vi "ErrorLogVI.vi"(8 "Error In":errorcluster, 11 "Station":string) -> ()   [LabVIEW 2017]
doc: "This VI log's Error to ErrLog.txt File.\nPath:- C:/.../Documents/VisionInsp folder in PC.\nChange Folder name If you want to save Error Log into Another Folder."
uses:
  <vilib>/Utility/sysdir.llb/System Directory Type.ctl
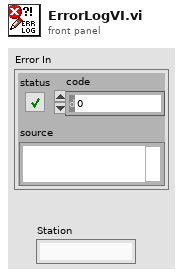
[diagram p1: front panel]
types:
  T1 = enum16{"open", "replace", "create", "open or create", "replace or create", "replace or create with confirmation"}
  T2 = typedef "System Directory Type.ctl" = i32
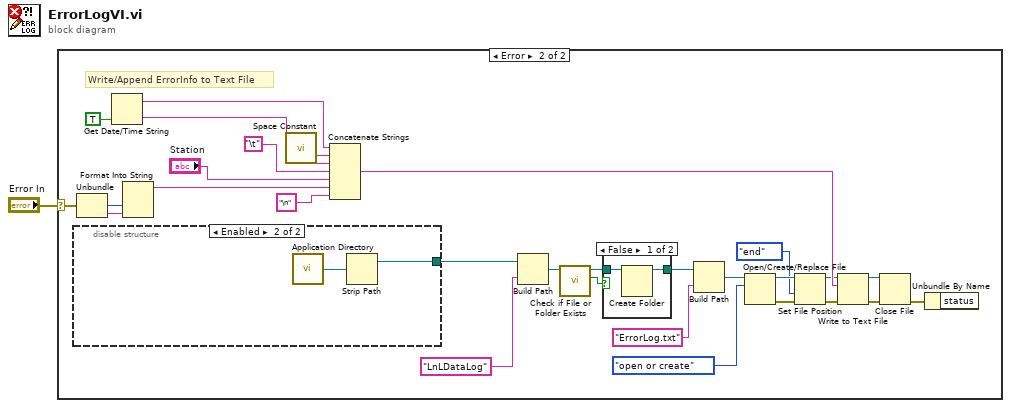
[diagram p0: block diagram]
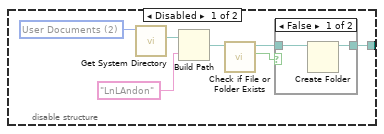
[diagram p3: hidden frame]
diagram:
  n1 = case shown="Error" "Error In" {
    selector: "Error In" -> [_ w4]
    frame No Error {
    }
    frame Error {
      # "Write/Append ErrorInfo to Text File"
      n2 = disable-structure shown="Enabled" {
        disable-tunnel: [w31 w41] -> w12
        frame Disabled {
          w37 = T2 2 items=["User Home"=0, "User Desktop"=1, "User Documents"=2, "User Application Data"=3, "User Preferences"=4, "User Temporary"=5, "Public Documents"=6, "Public Application Data"=7, "Public Preferences"=8, "Public Cache"=13, "System Core Libraries"=9, "System Installed Libraries"=10, "Application Files"=11, "Boot Volume Root"=12] ("system directory type")
          n3 = call <vilib>:"Get System Directory.vi"("system directory type"=w37) -> ("system directory"=w36:path)  [unwired: 10 in]
          n4 = Build Path(base path=w36, name or relative path="LnLAndon" ("Folder Name")) -> (appended path=w34:path)
          n5 = call <vilib>:"Check if File or Folder Exists.vi"("path"=w34) -> ("file or folder exists?"=w33:bool, "dup path"=w32:path)  [unwired: 8 in, 1 out]
          n6 = case shown="False" w33 {
            tunnel: w32 -> [w39 w40]
            tunnel: [w38 w40] -> w31
            frame False {
              n7 = Create Folder(path (use dialog)=w39) -> (created path=w38:path)  [unwired: 2 in, 2 out]
            }
            frame True {
            }
          }
        }
        frame Enabled {
          n8 = call <vilib>:"Application Directory.vi"() -> ("Application Directory"=w42:path)
          n9 = Strip Path(path=w42) -> (stripped path=w41:path)  [unwired: 1 out]
        }
      }
      n10 = Unbundle(w4) -> ("code"=w6:i32, "source"=w5:string)  [unwired: 1 out]
      n11 = Get Date/Time String(want seconds? (F)=TRUE) -> (date string=w17:string, time string=w29:string)  [unwired: 2 in]
      n12 = Format Into String(w6, w5) -> (resulting string=w18:string)  [unwired: 3 in, 1 out]
      n13 = call <vilib>:"Space Constant.vi"() -> ("String"=w15:string)
      n14 = Concatenate Strings(w17, w15, w29, "\t", "Station", w18, "\n") -> (w27:string)
      n15 = Build Path(base path=w12, name or relative path="LnLDataLog") -> (appended path=w8:path)
      n16 = call <vilib>:"Check if File or Folder Exists.vi"("path"=w8) -> ("file or folder exists?"=w9:bool, "dup path"=w10:path)  [unwired: 8 in, 1 out]
      n17 = case shown="False" w9 {
        tunnel: w10 -> [w44 w45]
        tunnel: [w43 w45] -> w7
        frame False {
          n18 = Create Folder(path (use dialog)=w44) -> (created path=w43:path)  [unwired: 2 in, 2 out]
        }
        frame True {
        }
      }
      n19 = Build Path(base path=w7, name or relative path="ErrorLog.txt") -> (appended path=w19:path)
      n20 = Open/Create/Replace File(file path (use dialog)=w19, operation (0:open)=T1."open or create") -> (refnum out=w26:refnum<file>, error out=w25:errorcluster)  [unwired: 4 in, 1 out]
      n21 = Set File Position(refnum=w26, from (0:start)=enum16{"start", "end", "current"}."end", error in=w25) -> (refnum out=w21:refnum<file>, error out=w22:errorcluster)  [unwired: 1 in]
      n22 = Write to Text File(file (use dialog)=w21, text=w27, error in=w22) -> (refnum out=w14:refnum<file>, error out=w13:errorcluster)  [unwired: 1 in, 1 out]
      n23 = Close File(refnum=w14, error in=w13) -> (error out=w3:errorcluster)  [unwired: 1 out]
      n24 = Unbundle By Name(w3) -> ()  [unwired: 1 out]
    }
  }
